vi "外观 1.vi"(0 "Data In":T4 caption="数据输入", 2 "Display State In":T2 caption="显示状态输入", 3 "Container State":T3 caption="容器状态") -> (6 "Data Out":T4 caption="数据输出", 7 "Display State Out":T2 caption="显示状态输出", 8 "Action":T1 caption="动作")   [LabVIEW 2016, in "总磷氨氮运行状态.xctl"]
uses:
  <vilib>/_xctls/Container State.ctl
  <vilib>/_xctls/Action.ctl
  <vilib>/_xctls/XControlSupport.lvlib
panel:
  out "运行参数":string
  out "故障信息":string
  out "告警信息":string
  out "测量模式":string
  out "工作状态":string
  out "仪器时间":string
  # "运行参数:"
  # "仪器时间:"
  # "工作状态:"
  # "测量模式:"
  # "告警信息:"
  # "故障信息:"
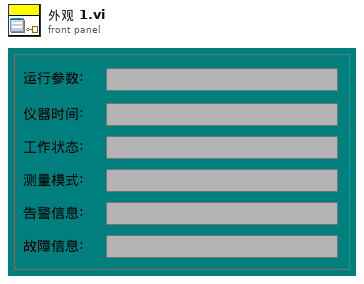
[diagram p1: front panel]
types:
  T1 = typedef "XControlSupport.lvlib/Action.ctl" = cluster{"Data Changed?":bool, "State Changed?":bool, "Action Name":string}
  T2 = typedef "总磷氨氮运行状态.xctl/状态 2.ctl" = cluster{"Numeric":dbl}
  T3 = typedef "XControlSupport.lvlib/Container State.ctl" = cluster{"Indicator?":bool, "Run Mode?":bool, " Refnum":refnum<vi>}
  T4 = typedef "总磷氨氮运行状态.xctl/数据 1.ctl" = cluster{"系统时间":timestamp, "工作状态":enum16{"空闲", "水样测试", "标样核查", "零点核查", "跨度核查", "空白测试", "平行样测试", "加标回收", "空白校准", "标样校准", "初始化（清洗）"}, "测量模式":enum16{"待机", "连续模式", "周期模式", "定点模式", "受控模式", "手动模式"}, "告警代码":enum16{"无告警", "缺试剂告警", "缺水样告警", "缺蒸馏水告警", "缺标液告警", "仪表漏液告警", "标定异常告警", "超量程告警", "加热异常", "低试剂预警", "超上限告警", "超下限告警", "仪表内部其他异常", "滴定异常告警", "电极异常告警", "量程切换告警", "参数设置告警", "PH电极电位异常", "电导率电极异常", "浊度光度异常", "溶解氧电极异常", "溶解氧光强异常", "温度异常告警", "PH异常告警", "溶解氧异常告警", "电导率异常告警", "浊度异常告警", "叶绿素异常告警", "藻密度异常告警", "蓝绿藻异常告警", "ORP异常告警", "氨氮异常告警", "清洁刷异常告警", "SD卡异常告警", "蓝牙异常告警", "Wifi异常告警", "流程异常告警"}, "故障代码":enum16{"无故障", "电机故障", "温度故障", "通讯故障", "滴定故障"}, "日志代码":u16, "软件版本":u16, "F0":sgl, "F1":sgl, "F2":sgl, "F3":sgl, "T":sgl, "H":sgl, "id":u16, "flowid":u16, "量程":u16, "总磷控温温度1":sgl, "营养盐控温温度2":sgl, "ADC":sgl}
  T5 = enum16{"空闲", "水样测试", "标样核查", "零点核查", "跨度核查", "空白测试", "平行样测试", "加标回收", "空白校准", "标样校准", "初始化（清洗）"}
  T6 = enum16{"待机", "连续模式", "周期模式", "定点模式", "受控模式", "手动模式"}
  T7 = enum16{"无告警", "缺试剂告警", "缺水样告警", "缺蒸馏水告警", "缺标液告警", "仪表漏液告警", "标定异常告警", "超量程告警", "加热异常", "低试剂预警", "超上限告警", "超下限告警", "仪表内部其他异常", "滴定异常告警", "电极异常告警", "量程切换告警", "参数设置告警", "PH电极电位异常", "电导率电极异常", "浊度光度异常", "溶解氧电极异常", "溶解氧光强异常", "温度异常告警", "PH异常告警", "溶解氧异常告警", "电导率异常告警", "浊度异常告警", "叶绿素异常告警", "藻密度异常告警", "蓝绿藻异常告警", "ORP异常告警", "氨氮异常告警", "清洁刷异常告警", "SD卡异常告警", "蓝牙异常告警", "Wifi异常告警", "流程异常告警"}
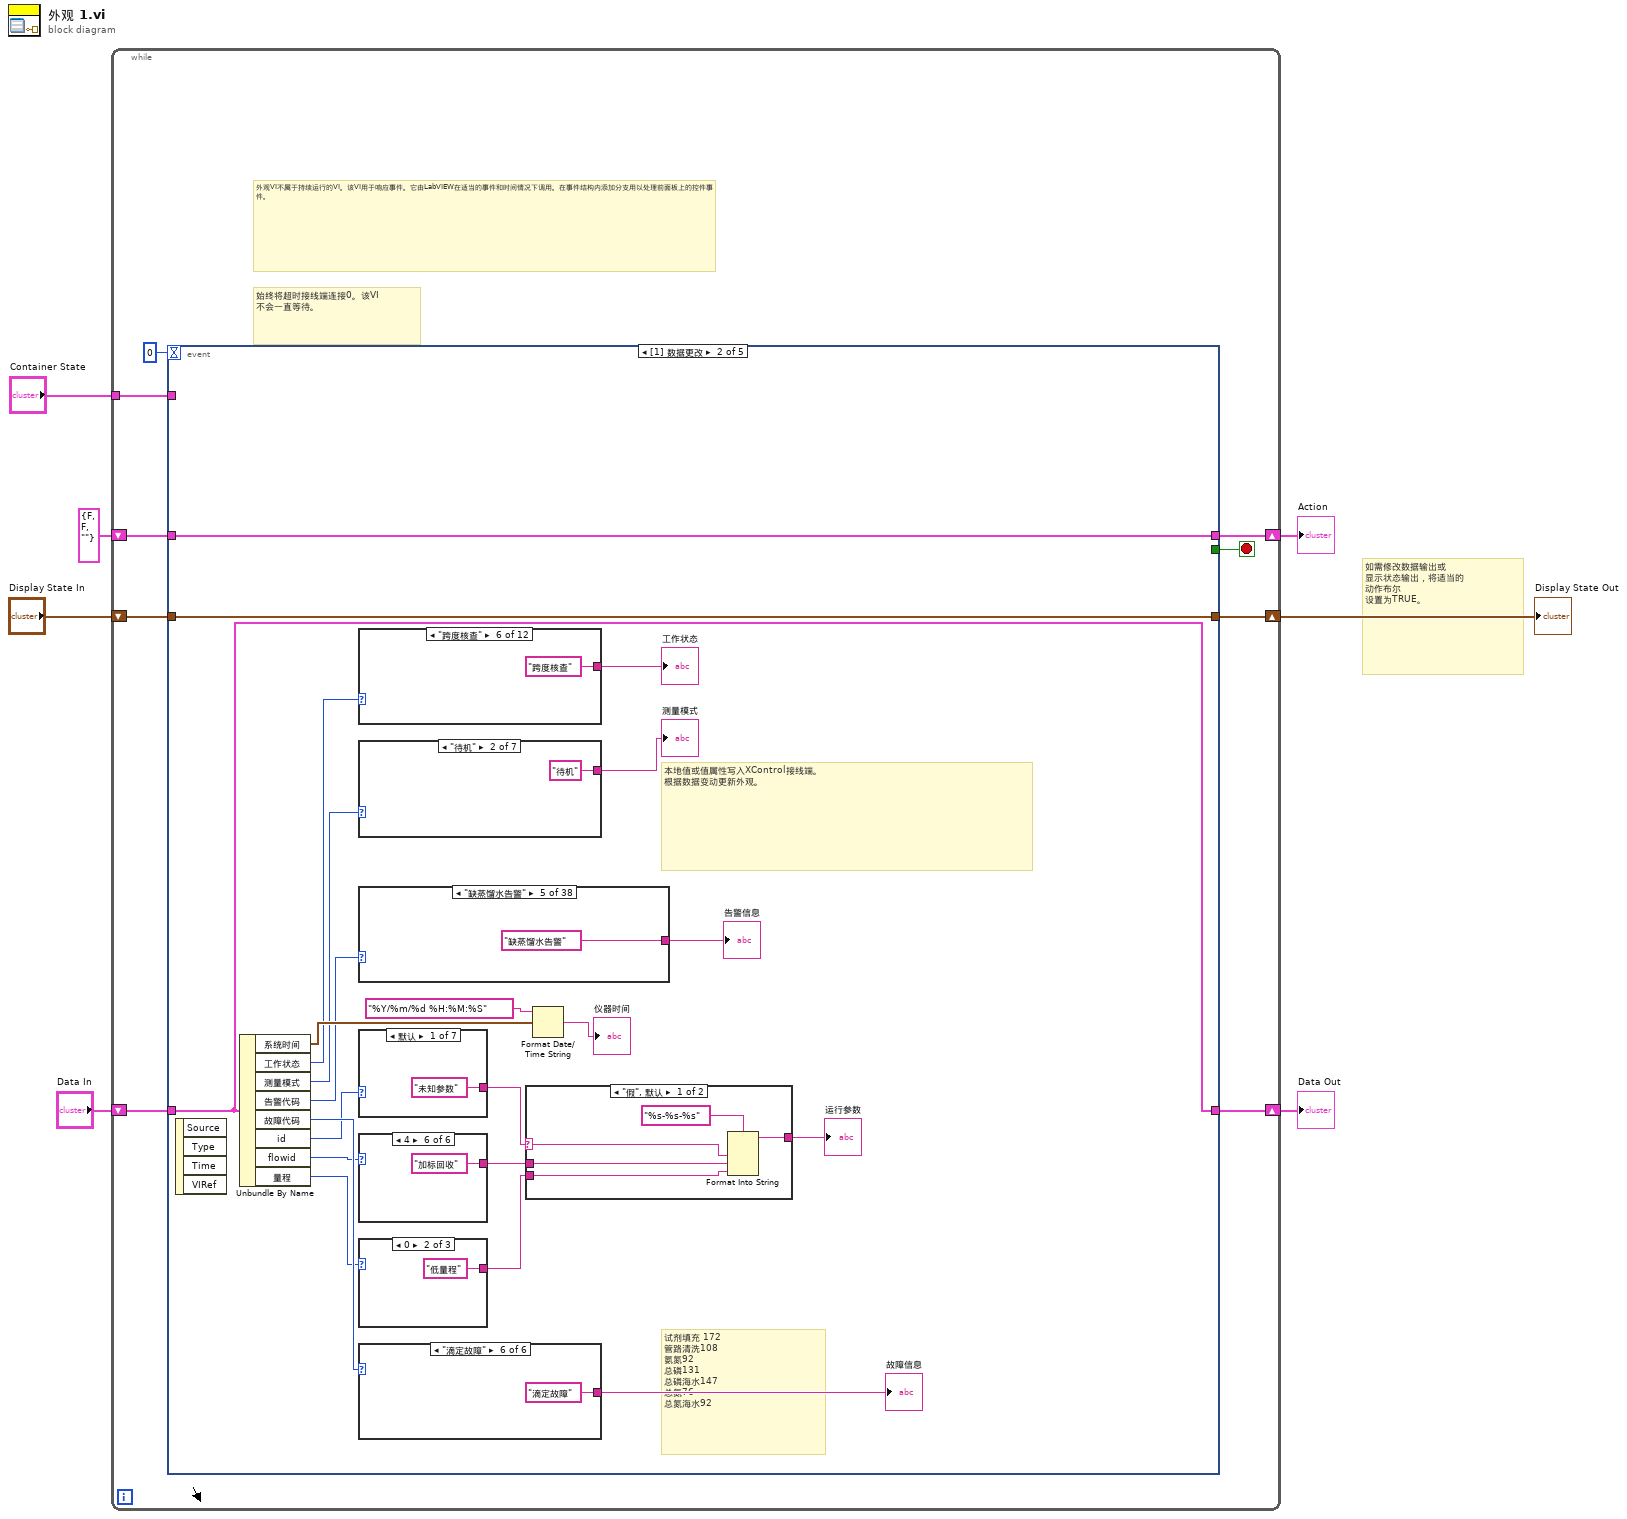
[diagram p0: block diagram]
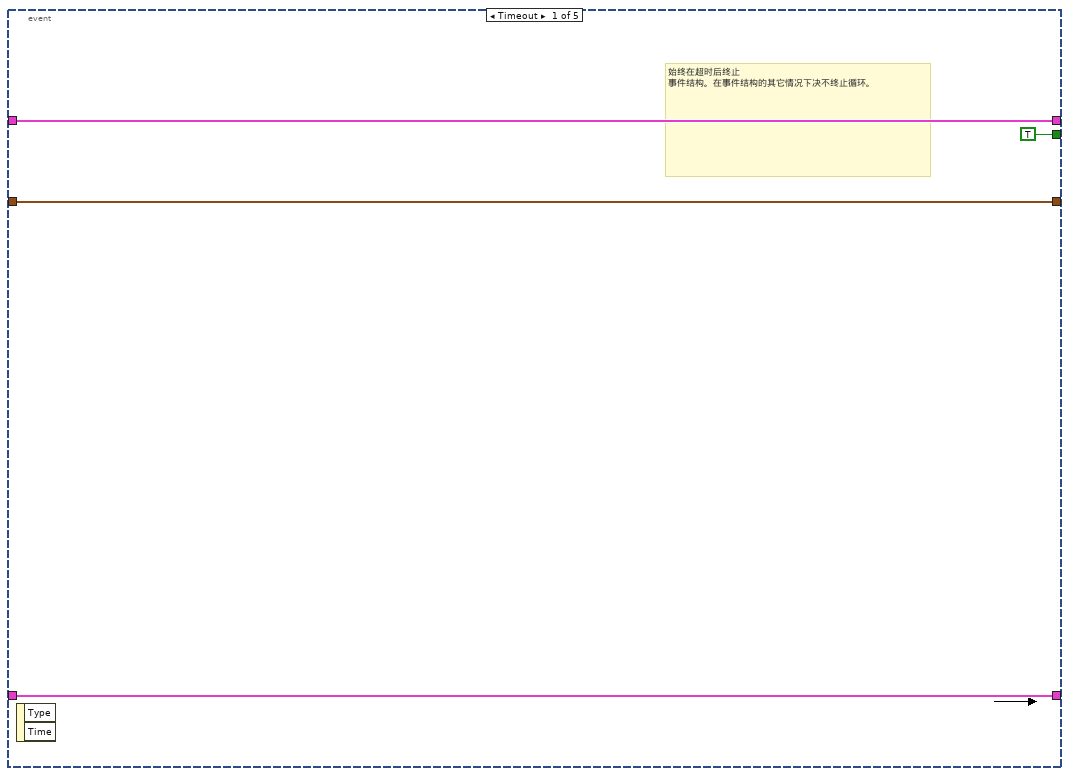
[diagram p2: hidden frame]
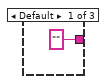
[diagram p4: hidden frame]
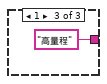
[diagram p5: hidden frame]
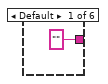
[diagram p6: hidden frame]
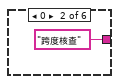
[diagram p7: hidden frame]
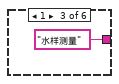
[diagram p8: hidden frame]
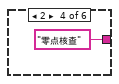
[diagram p9: hidden frame]
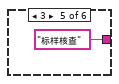
[diagram p10: hidden frame]
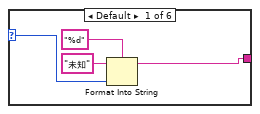
[diagram p11: hidden frame]
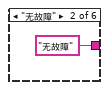
[diagram p12: hidden frame]
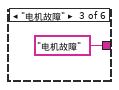
[diagram p13: hidden frame]
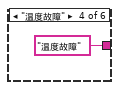
[diagram p14: hidden frame]
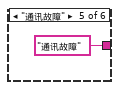
[diagram p15: hidden frame]
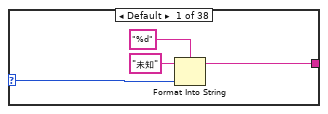
[diagram p16: hidden frame]
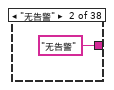
[diagram p17: hidden frame]
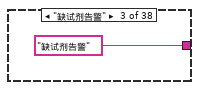
[diagram p18: hidden frame]
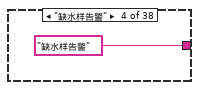
[diagram p19: hidden frame]
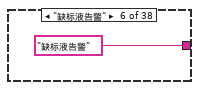
[diagram p20: hidden frame]
diagram:
  # "如需修改数据输出或\n显示状态输出，将适当的\n动作布尔\n设置为TRUE。"
  n1 = while {
    shift-right: [w15] -> w4
    shift-left: "Display State In" -> [w16]
    tunnel: "Container State" -> [w12]
    shift-right: [w10] -> w7
    shift-left: "Data In" -> [w11]
    shift-right: [w8] -> w2
    shift-left: T1 {"Data Changed?"=FALSE, "State Changed?"=FALSE, "Action Name"=""} ("Action") -> [w9]
    stop <- w14 stop-if-true
    # "外观VI不属于持续运行的VI。该VI用于响应事件。它由LabVIEW在适当的事件和时间情况下调用。在事件结构内添加分支用以处理前面板上的控件事件。"
    # "始终将超时接线端连接0。该VI\n不会一直等待。"
    n2 = event shown="[1] 数据更改" {
      selector: _ -> [_ _ _ _ _]
      dyn-events: _ -> [_ _ _ _ _]
      timeout: 0 -> [_ _ _ _ _]
      tunnel: w16 -> [w18 w41 w140 w143 w147]
      tunnel: [w18 w41 w140 w143 w147] -> w15
      tunnel: [TRUE _ _ _ _] -> w14
      tunnel: w12 -> [_ _ _ w144 w148]
      tunnel: w11 -> [w17 w39 w139 w142 w146]
      tunnel: [w17 w39 w139 w142 w146] -> w10
      tunnel: [w19 w40 w138 w141 w145] -> w8
      tunnel: w9 -> [w19 w40 w138 w141 w145]
      event Timeout {
        # "始终在超时后终止\n事件结构。在事件结构的其它情况下决不终止循环。"
        n3 = event-data() -> ()  [unwired: 1 in, 2 out]
      }
      event Data Change {
        # "试剂填充 172 \n管路清洗108\n氨氮92\n总磷131\n总磷海水147\n总氮76\n总氮海水92"
        # "本地值或值属性写入XControl接线端。\n根据数据变动更新外观。"
        n4 = event-data() -> ()  [unwired: 1 in, 4 out]
        n5 = Unbundle By Name(w39) -> ("系统时间"=w37:timestamp, "工作状态"=w35:T5, "测量模式"=w33:T6, "告警代码"=w31:T7, "故障代码"=w29:enum16{"无故障", "电机故障", "温度故障", "通讯故障", "滴定故障"}, "id"=w27:u16, "flowid"=w26:u16, "量程"=w25:u16)
        n6 = case shown="\"跨度核查\"" w35 {
          selector: w35 -> [w116 _ _ _ _ _ _ _ _ _ _ _]
          tunnel: [w117 "空闲" ("工作状态") "水样测量" ("工作状态") "标样核查" ("工作状态") "零点核查" ("工作状态") "跨度核查" ("工作状态") "空白测试" ("工作状态") "平行样测试" ("工作状态") "加标回收" ("工作状态") "空白校准" ("工作状态") "标样校准" ("工作状态") "初始化" ("工作状态")] -> w34
          frame Default {
            n7 = Format Into String(format string="%d" ("格式字符串"), initial string="未知" ("工作状态"), w116) -> (resulting string=w117:string)  [unwired: 1 in, 1 out]
          }
          frame "空闲" {
          }
          frame "水样测试" {
          }
          frame "标样核查" {
          }
          frame "零点核查" {
          }
          frame "跨度核查" {
          }
          frame "空白测试" {
          }
          frame "平行样测试" {
          }
          frame "加标回收" {
          }
          frame "空白校准" {
          }
          frame "标样校准" {
          }
          frame "初始化（清洗）" {
          }
        }
        "工作状态" <- w34
        n8 = case shown="\"待机\"" w33 {
          selector: w33 -> [w106 _ _ _ _ _ _]
          tunnel: [w107 "待机" "连续模式" "周期模式" "定点模式" "受控模式" "手动模式"] -> w32
          frame Default {
            n9 = Format Into String(format string="%d" ("格式字符串"), initial string="未知" ("工作状态"), w106) -> (resulting string=w107:string)  [unwired: 1 in, 1 out]
          }
          frame "待机" {
          }
          frame "连续模式" {
          }
          frame "周期模式" {
          }
          frame "定点模式" {
          }
          frame "受控模式" {
          }
          frame "手动模式" {
          }
        }
        "测量模式" <- w32
        n10 = case shown="\"缺蒸馏水告警\"" w31 {
          selector: w31 -> [w66 _ _ _ _ _ _ _ _ _ _ _ _ _ _ _ _ _ _ _ _ _ _ _ _ _ _ _ _ _ _ _ _ _ _ _ _ _]
          tunnel: [w65 "无告警" "缺试剂告警" "缺水样告警" "缺蒸馏水告警" "缺标液告警" "仪表漏液告警" "标定异常告警" "超量程告警" "加热异常" "低试剂预警" "超上限告警" "超下限告警" "仪表内部其他异常" "滴定异常告警" "电极异常告警" "量程切换告警" "参数设置告警" "PH电极电位异常" "电导率电极异常" "浊度光度异常" "溶解氧电极异常" "溶解氧光强异常" "温度异常告警" "PH异常告警" "溶解氧异常告警" "电导率异常告警" "浊度异常告警" "叶绿素异常告警" "藻密度异常告警" "蓝绿藻异常告警" "ORP异常告警" "氨氮异常告警" "清洁刷异常告警" "SD卡异常告警" "蓝牙异常告警" "WiFi异常告警" "流程异常告警"] -> w30
          frame Default {
            n11 = Format Into String(format string="%d" ("格式字符串"), initial string="未知" ("工作状态"), w66) -> (resulting string=w65:string)  [unwired: 1 in, 1 out]
          }
          frame "无告警" {
          }
          frame "缺试剂告警" {
          }
          frame "缺水样告警" {
          }
          frame "缺蒸馏水告警" {
          }
          frame "缺标液告警" {
          }
          frame "仪表漏液告警" {
          }
          frame "标定异常告警" {
          }
          frame "超量程告警" {
          }
          frame "加热异常" {
          }
          frame "低试剂预警" {
          }
          frame "超上限告警" {
          }
          frame "超下限告警" {
          }
          frame "仪表内部其他异常" {
          }
          frame "滴定异常告警" {
          }
          frame "电极异常告警" {
          }
          frame "量程切换告警" {
          }
          frame "参数设置告警" {
          }
          frame "PH电极电位异常" {
          }
          frame "电导率电极异常" {
          }
          frame "浊度光度异常" {
          }
          frame "溶解氧电极异常" {
          }
          frame "溶解氧光强异常" {
          }
          frame "温度异常告警" {
          }
          frame "PH异常告警" {
          }
          frame "溶解氧异常告警" {
          }
          frame "电导率异常告警" {
          }
          frame "浊度异常告警" {
          }
          frame "叶绿素异常告警" {
          }
          frame "藻密度异常告警" {
          }
          frame "蓝绿藻异常告警" {
          }
          frame "ORP异常告警" {
          }
          frame "氨氮异常告警" {
          }
          frame "清洁刷异常告警" {
          }
          frame "SD卡异常告警" {
          }
          frame "蓝牙异常告警" {
          }
          frame "Wifi异常告警" {
          }
          frame "流程异常告警" {
          }
        }
        "告警信息" <- w30
        n12 = case shown="默认" w27 {
          tunnel: ["未知参数" ("运行参数") "总氮" ("运行参数") "氨氮" ("运行参数") "总磷海水" ("运行参数") "管路清洗" ("运行参数") "试剂填充" ("运行参数") "总磷" ("运行参数")] -> w24
          frame Default {
          }
          frame 76 {
          }
          frame 92 {
          }
          frame 147 {
          }
          frame 108 {
          }
          frame 172 {
          }
          frame 131 {
          }
        }
        n13 = case shown="4" w26 {
          tunnel: ["" ("字符串") "跨度核查" ("字符串") "水样测量" ("字符串") "零点核查" ("字符串") "标样核查" ("字符串") "加标回收" ("字符串")] -> w22
          frame Default {
          }
          frame 0 {
          }
          frame 1 {
          }
          frame 2 {
          }
          frame 3 {
          }
          frame 4 {
          }
        }
        n14 = case shown="0" w25 {
          tunnel: ["" ("字符串") "低量程" ("字符串") "高量程" ("字符串")] -> w21
          frame Default {
          }
          frame 0 {
          }
          frame 1 {
          }
        }
        n15 = case shown="\"滴定故障\"" w29 {
          selector: w29 -> [w57 _ _ _ _ _]
          tunnel: [w56 "无故障" "电机故障" "温度故障" "通讯故障" "滴定故障"] -> w28
          frame Default {
            n16 = Format Into String(format string="%d" ("格式字符串"), initial string="未知" ("工作状态"), w57) -> (resulting string=w56:string)  [unwired: 1 in, 1 out]
          }
          frame "无故障" {
          }
          frame "电机故障" {
          }
          frame "温度故障" {
          }
          frame "通讯故障" {
          }
          frame "滴定故障" {
          }
        }
        "故障信息" <- w28
        n17 = case shown="\"假\", 默认" w24 {
          selector: w24 -> [w44 _]
          tunnel: [w45 _] -> w23
          tunnel: w22 -> [w43 _]
          tunnel: w21 -> [w42 _]
          frame "假", Default {
            n18 = Format Into String(format string="%s-%s-%s" ("格式字符串"), w44, w43, w42) -> (resulting string=w45:string)  [unwired: 2 in, 1 out]
          }
          frame "未知参数" {
          }
        }
        "运行参数" <- w23
        n19 = Format Date/Time String(time format string (%c)="%Y/%m/%d %H:%M:%S" ("时间格式字符串(%c)"), seconds (now)=w37) -> (date/time string=→"仪器时间":string)  [unwired: 1 in]
      }
      event Display State Change {
        # "拖放该XControl的新实例、复制、撤消操作或者在XControl内执行自定义属性或方法均可改变显示状态。更新相应外观。"
        n20 = event-data() -> ()  [unwired: 1 in, 4 out]
      }
      event Direction Change {
        # "XControl的方向由输入控件转换为显示控件，反之亦然。更新相应外观。"
        n21 = event-data() -> ()  [unwired: 1 in, 4 out]
        n22 = Unbundle By Name(w144) -> ()  [unwired: 1 out]
      }
      event Exec State Change {
        # "包含该XControl的VI已从编辑模式切换至运行模式，反之亦然。\n相应的更新外观。"
        # "分别处理编辑模式和\n运行模式"
        n23 = event-data() -> ()  [unwired: 1 in, 4 out]
        n24 = Unbundle By Name(w148) -> ()  [unwired: 1 out]
      }
    }
  }
  "Display State Out" <- w4
  "Data Out" <- w7
  "Action" <- w2
